vi "Add Caption to All Controls.vi"() -> ()   [LabVIEW 2017, in "Localization.lvlib"]
uses:
  Localization.lvlib
  Control Info/Control Info.lvclass
panel:
  in  "vi path":path
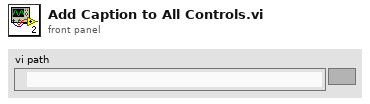
[diagram p1: front panel]
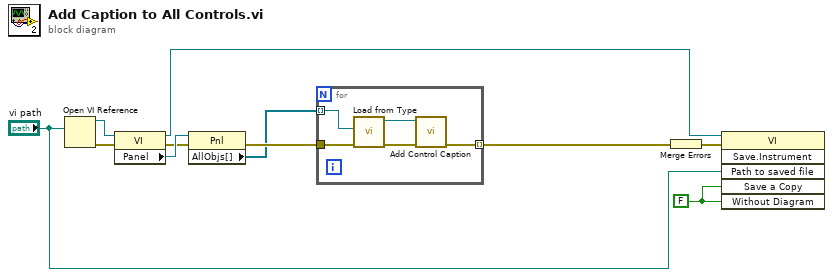
[diagram p0: block diagram]
diagram:
  w1 = FALSE ("Without Diagram")
  n1 = Open VI Reference(vi path="vi path") -> (vi reference=w8:refnum<vi>, error out=w9:errorcluster)  [unwired: 5 in]
  n2 = property class="VI"(reference=w8, error in=w9) -> (reference out=w3:refnum<vi>, error out=w10:errorcluster, "Panel"=w11:refnum<vi>)
  n3 = property class="Pnl"(reference=w11, error in=w10) -> (error out=w7:errorcluster, "AllObjs[]"=w6:refnum<vi>[])  [unwired: 1 out]
  n4 = for {
    tunnel: w6 -> [w16] mode=indexing
    tunnel: w7 -> [w15]
    tunnel: [w12] -> w4 mode=indexing
    n5 = call "Load from Type.vi"("error in (no error)"=w15, "Control Reference"=w16) -> ("error out"=w14:errorcluster, "Control Info out"=w13:refnum<class "Control Info.lvclass">)  [unwired: 8 in]
    n6 = call-dynamic "Add Control Caption.vi"("error in (no error)"=w14, "Control Info in"=w13) -> ("error out"=w12:errorcluster)  [unwired: 8 in, 1 out]
  }
  n7 = Merge Errors(w4) -> (w5:errorcluster)
  n8 = invoke class="VI" method="Save.Instrument"(reference=w3, error in=w5, "Path to saved file"="vi path", "Save a Copy"=w1, "Without Diagram"=w1) -> ()  [unwired: 1 in, 6 out]
